vi "Program for Jack (JRD edits).vi"(8 "error in":errorcluster, 11 "Version":string="2.0.8.1007") -> (0 "error out":errorcluster)   [LabVIEW 2013]
uses:
  <resource>/Framework/Providers/Wirebird Labs LLC/Deploy/Support/Update Service/Deploy-UpdateService.lvclass
panel:
  in  "stop":bool
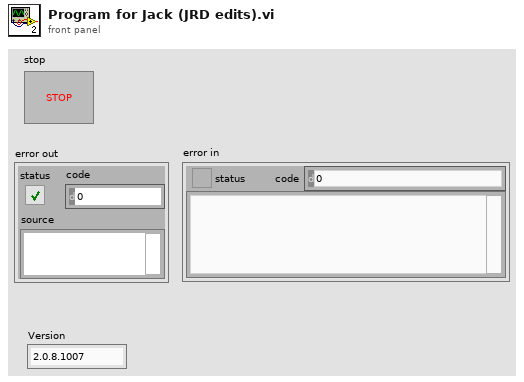
[diagram p1: front panel]
types:
  T1 = typedef "Deploy-UpdateService.lvclass/Deploy-UpdateService-Event-Dialog.ctl" = enum16{"Dialog Opened", "Dialog Closed", "Dialog Dismissed"}
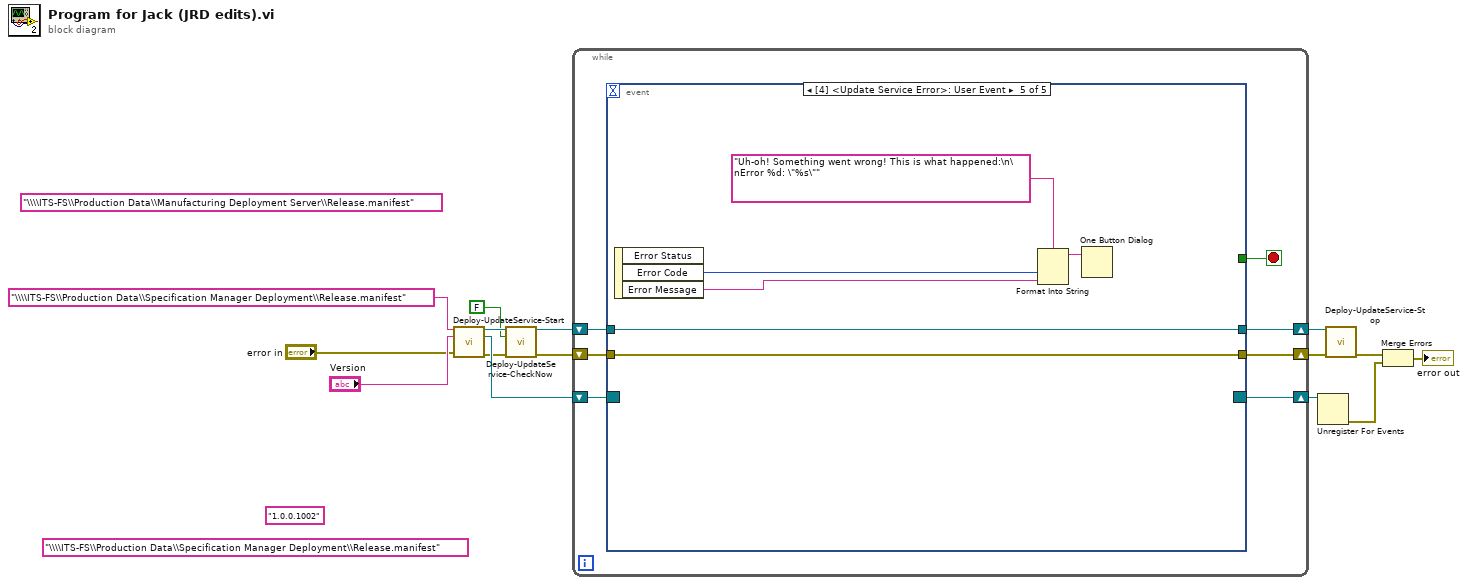
[diagram p0: block diagram]
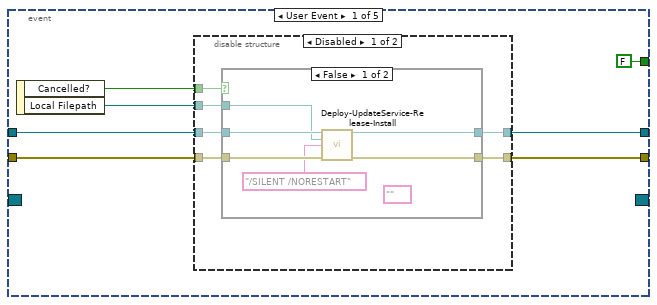
[diagram p2: hidden frame]
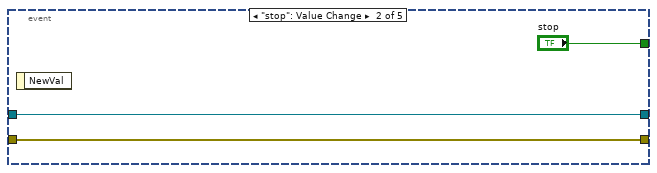
[diagram p5: hidden frame]
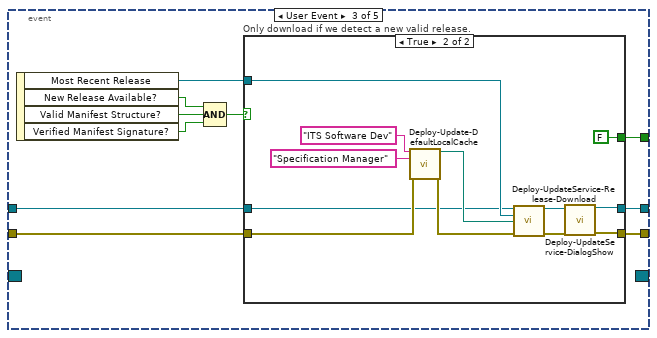
[diagram p6: hidden frame]
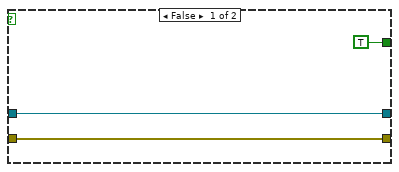
[diagram p7: hidden frame]
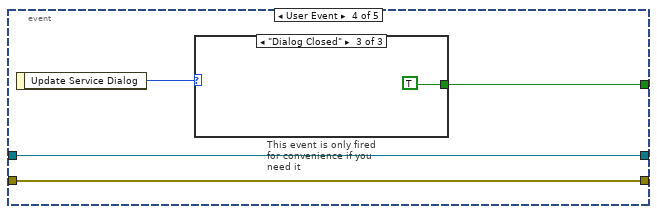
[diagram p8: hidden frame]
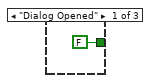
[diagram p9: hidden frame]
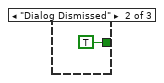
[diagram p10: hidden frame]
diagram:
  (unwired) "\\\\ITS-FS\\Production Data\\Manufacturing Deployment Server\\Release.manifest" ("Manifest URI")
  (unwired) "1.0.0.1002" ("Current Release Version")
  (unwired) "\\\\ITS-FS\\Production Data\\Specification Manager Deployment\\Release.manifest" ("Manifest URI")
  n1 = call <resource>:"Deploy-UpdateService-Start.vi"("Manifest URI"="\\\\ITS-FS\\Production Data\\Specification Manager Deployment\\Release.manifest", "Current Release Version"="Version", "error in"="error in") -> ("Update Service"=w14:refnum<class "Deploy-UpdateService.lvclass">, "Update Service Event Registration"=w15:refnum<event-registration>, "error out"=w13:errorcluster)  [unwired: 10 in]
  n2 = call <resource>:"Deploy-UpdateService-CheckNow.vi"("Update Service"=w14, "Show UI?"=FALSE, "error in"=w13) -> ("Update Service out"=w12:refnum<class "Deploy-UpdateService.lvclass">, "error out"=w11:errorcluster)  [unwired: 11 in]
  n3 = while {
    shift-right: [w21] -> w6
    shift-left: w11 -> [w19]
    shift-right: [w17] -> w9
    shift-left: w15 -> [w22]
    shift-right: [w16] -> w7
    shift-left: w12 -> [w20]
    stop <- w18 stop-if-true
    n4 = event shown="[4] <Update Service Error>: User Event" {
      selector: w22 -> [_ _ _ _ _]
      dyn-events: [_ _ _ _ _] -> w17
      timeout: _ -> [_ _ _ _ _]
      tunnel: w20 -> [w29 w46 w58 w77 w85]
      tunnel: w19 -> [w28 w47 w56 w76 w84]
      tunnel: [w24 w47 w55 w76 w84] -> w21
      tunnel: [FALSE ("stop") "stop" w49 w74 _] -> w18
      tunnel: [w25 w46 w50 w77 w85] -> w16
      event User Event {
        n5 = event-data() -> ("Cancelled?"=w23:bool, "Local Filepath"=w27:path)  [unwired: 1 in]
        n6 = disable-structure shown="Disabled" {
          disable-tunnel: w29 -> [w35 w44]
          disable-tunnel: w28 -> [w34 w45]
          disable-tunnel: w27 -> [w33 _]
          disable-tunnel: [w32 w44] -> w25
          disable-tunnel: [w31 w45] -> w24
          disable-tunnel: w23 -> [w30 _]
          frame Disabled {
            n7 = case shown="False" w30 {
              tunnel: w35 -> [w41 w43]
              tunnel: w34 -> [w40 w42]
              tunnel: w33 -> [w39 _]
              tunnel: [w38 w43] -> w32
              tunnel: [w37 w42] -> w31
              frame False {
                (unwired) "" ("Installer Command Line Parameters")
                n8 = call <resource>:"Deploy-UpdateService-Release-Install.vi"("Update Service"=w41, "Downloaded Release Filepath"=w39, "Installer Command Line Parameters"="/SILENT /NORESTART", "error in"=w40) -> ("Update Service out"=w38:refnum<class "Deploy-UpdateService.lvclass">, "error out"=w37:errorcluster)  [unwired: 10 in]
              }
              frame True {
              }
            }
          }
          frame Enabled {
          }
        }
      }
      event "stop": Value Change {
        n9 = event-data() -> ()  [unwired: 1 in, 1 out]
      }
      event User Event {
        n10 = event-data() -> ("Most Recent Release"=w57:refnum<class "Deploy-Release.lvclass">, "New Release Available?"=w54:bool, "Valid Manifest Structure?"=w53:bool, "Verified Manifest Signature?"=w52:bool)  [unwired: 1 in]
        n11 = Compound Arithmetic op=AND(w54, w53, w52) -> (w51:bool)
        n12 = case "Only download if we detect a new valid release." shown="True" w51 {
          tunnel: w58 -> [w61 w67]
          tunnel: w57 -> [_ w71]
          tunnel: w56 -> [w60 w70]
          tunnel: [w60 w62] -> w55
          tunnel: [w61 w63] -> w50
          tunnel: [TRUE FALSE] -> w49
          frame False {
          }
          frame True {
            n13 = call <resource>:"Deploy-Update-DefaultLocalCache.vi"("Publisher (Organization)"="ITS Software Dev", "Application (Product Name)"="Specification Manager", "error in"=w70) -> ("Default Local Cache Directory"=w69:path, "error out"=w68:errorcluster)  [unwired: 11 in]
            n14 = call <resource>:"Deploy-UpdateService-Release-Download.vi"("Update Service"=w67, "Release to Download"=w71, "Local Download Cache"=w69, "error in"=w68) -> ("Update Service out"=w65:refnum<class "Deploy-UpdateService.lvclass">, "error out"=w64:errorcluster)  [unwired: 10 in]
            n15 = call <resource>:"Deploy-UpdateService-DialogShow.vi"("Update Service"=w65, "error in"=w64) -> ("Update Service out"=w63:refnum<class "Deploy-UpdateService.lvclass">, "error out"=w62:errorcluster)  [unwired: 12 in]
          }
        }
      }
      event User Event {
        n16 = event-data() -> ("Update Service Dialog"=w75:T1)  [unwired: 1 in]
        n17 = case "This event is only fired for convenience if you need it" shown="\"Dialog Closed\"" w75 {
          tunnel: [FALSE TRUE TRUE] -> w74
          frame "Dialog Opened" {
          }
          frame "Dialog Dismissed" {
          }
          frame "Dialog Closed" {
          }
        }
      }
      event User Event {
        n18 = event-data() -> ("Error Code"=w83:i32, "Error Message"=w82:string)  [unwired: 1 in, 1 out]
        n19 = Format Into String(format string="Uh-oh! Something went wrong! This is what happened:\n\nError %d: \"%s\"", w83, w82) -> (resulting string=w81:string)  [unwired: 2 in, 1 out]
        n20 = One Button Dialog(message=w81) -> ()  [unwired: 1 in, 1 out]
      }
    }
  }
  n21 = Unregister For Events(event registration refnum=w9) -> (error out=w8:errorcluster)  [unwired: 1 in]
  n22 = call <resource>:"Deploy-UpdateService-Stop.vi"("Update Service"=w7, "error in"=w6) -> ("error out"=w5:errorcluster)  [unwired: 13 in]
  n23 = Merge Errors(w5, w8) -> (→"error out":errorcluster)
